vi "Parse URL Pattern String.vi"(10 "Base URL String":string, 11 "Pattern String":string) -> (3 "Pattern":T1)   [LabVIEW 2020, in "Stream.lvlib"]
uses:
  Stream.lvlib
  URLPattern/URL Pattern Init.ctl
  URLPattern/URLPattern.lvclass
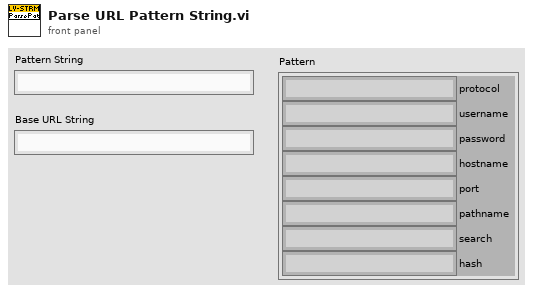
[diagram p1: front panel]
types:
  T1 = typedef "Stream.lvlib/URLPattern.lvclass/URL Pattern Init.ctl" = cluster{"protocol":string, "username":string, "password":string, "hostname":string, "port":string, "pathname":string, "search":string, "hash":string}
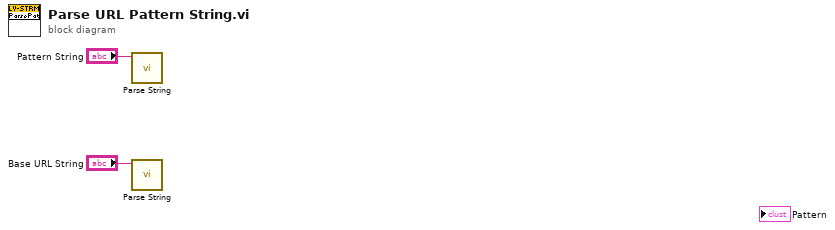
[diagram p0: block diagram]
diagram:
  n1 = call "Parse String.vi"("Pattern String"="Pattern String") -> ()  [unwired: 10 in, 1 out]
  n2 = call "Parse String.vi"("Pattern String"="Base URL String") -> ()  [unwired: 10 in, 1 out]
